vi "Idle Ref Image-Channel ctrls state.vi"() -> ()   [LabVIEW 2020]
uses:
  Typedefs/HW config states enum.ctl
  Typedefs/Channel control synergistic behaviour enum.ctl
  Global Variables/General Globals.vi
  Globals/gl_Windows Ctrl refs.vi
panel:
  out "error out":errorcluster
  in  "error in (no error)":errorcluster
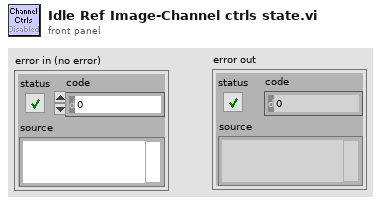
[diagram p1: front panel]
types:
  T1 = typedef "HW config states enum.ctl" = enum16{"Load from file", "Save to file", "Save backup", "Write all", "Read all", "Write XY stage settings", "Write DAQ FPGA settings", "Write Control FPGA settings", "Write Phys Channels", "Write System Config", "Write HW Config", "Save System Config", "Save HW Config", "Clear", "Compare from file"}
  T2 = typedef "Hardware Configuration settings.ctl" = cluster{"Dev. PC":bool, "Swap XY on stage":bool, "No of AOD":u8, "MC Supported":bool, "Axial MC":bool, "Computer MAC address":string, "Externalise Triggers":bool, "Trigger HW config":T3, "DAQmx Chan":T4, "XY stage available":bool, "XY Stage":T5, "Z stage available":bool, "Z Stage config cluster":T6, "Encoder available":bool, "Encoder":T7, "VidRec available":bool, "Cam VidRec":T8, "Laser Power Control HW config":T9, "Laser 1 available":bool, "Laser 1 config cluster":T10, "Prechirper 1 available":bool, "Prechirper 1 config cluster":T11, "Control system.FPGA available?":bool, "Control Sys. HW config":T12, "DAQ FPGA HW Config":T13, "PMT Voltage Range":T17}
  T3 = typedef "Triggers HW config.ctl" = cluster{"Available Device List":i32, "Device Address":string}
  T4 = typedef "DAQmx physical channels cluster.ctl" = cluster{"Pockels AO":tag, "Hard shutter AO":tag, "PMT AOs":tag, "Galvo AOs":tag, "Power meter AI":tag}
  T5 = typedef "XY Stage config cluster.ctl" = cluster{"COM port":refnum<visa-resource-name>, "Baudrate":i32, "Type":string}
  T6 = typedef "Z Stage config cluster.ctl" = cluster{"COM port":refnum<visa-resource-name>, "Baudrate":i32, "Type":string}
  T7 = typedef "Encoder config cluster.ctl" = cluster{"IP address":string, "Port":u16, "Wheel radius (cm)":dbl, "Encoder Trigger":tag}
  T8 = typedef "Cam VidRec HW config setup cluster.ctl" = cluster{"DO flag-Video record":tag, "DO flag-Trial start":tag}
  T9 = typedef "Laser Power Control HW config.ctl" = cluster{"Laser Power Control":string, "Laser Power Modulation Control":enum16{"NI", "FPGA"}}
  T10 = typedef "Laser 1 config cluster.ctl" = cluster{"COM port":refnum<visa-resource-name>, "Baud Rate":i32, "Type":string}
  T11 = typedef "PreChirper 1 config cluster.ctl" = cluster{"Type":string, "Baud Rate":i32, "COM port":refnum<visa-resource-name>}
  T12 = typedef "Control Sys HW config cluster.ctl" = cluster{"Control system.FPGA Type":enum16{"Virtex 5", "Virtex 7"}, "Control system.Network adapter name":string, "Control system.MAC address":string, "Control system.Ethernet Port":u32, "Control system.Ethernet Port Opened":bool}
  T13 = typedef "DAQ FPGA HW config cluster.ctl" = cluster{"FGPA Ref":T14, "Target":T15, "input card type":T16}
  T14 = typedef "FPGA Ref.ctl" = refnum<k20>
  T15 = typedef "nirio_resource_hc.ctl" = tag
  T16 = typedef "FPGA input type AC-DC.ctl" = enum16{"AC Card", "DC Card"}
  T17 = typedef "PMT Voltage Range.ctl" = cluster{"PMT Voltage Lower Limit":dbl, "PMT Voltage Upper Limit":dbl}
  T18 = typedef "Channel control synergistic behaviour enum.ctl" = enum16{"Left disabled-Right enabled", "Left enabled-Right disabled", "Both enabled"}
  T19 = typedef "Live window-ctrl refs.ctl" = cluster{"This VI":refnum<vi>, "Pane":refnum<vi>, "Show REF Image Left":refnum<vi>, "Show REF Image Right":refnum<vi>, "Snapshot":refnum<vi>, "Left Image Palette":refnum<vi>, "Right Image Palette":refnum<vi>, "Left Channel":refnum<vi>, "Right Channel":refnum<vi>, "Left image intensity":refnum<vi>, "Right image intensity":refnum<vi>, "Left Image Display":T20, "Right Image Display":T20, "Refresh rate ind (Hz)":refnum<vi>, "Acq rate ind (Hz)":refnum<vi>, "Stop (ind)":refnum<vi>}
  T20 = typedef "Image display ref.ctl" = refnum<vi>
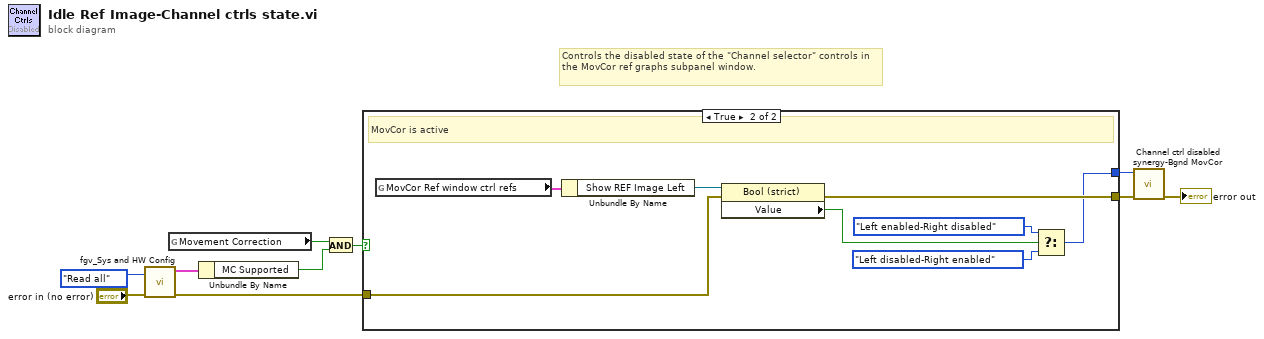
[diagram p0: block diagram]
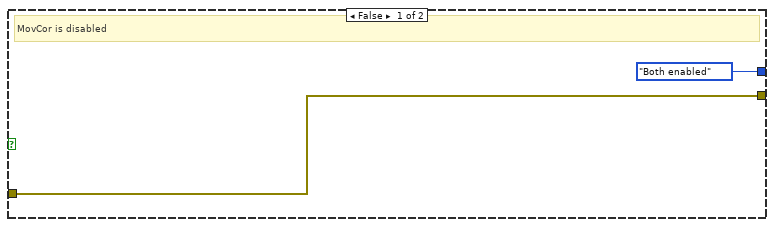
[diagram p2: hidden frame]
diagram:
  # "Controls the disabled state of the \"Channel selector\" controls in the MovCor ref graphs subpanel window."
  n1 = call "fgv_Sys and HW Config.vi"("Function"=HW_config_states_enum."Read all", "error in (no error)"="error in (no error)") -> ("error out"=w5:errorcluster, "Hardware Configuration OUT"=w10:T2)  [unwired: 7 in, 1 out]
  n2 = global read "General Globals.vi" "Movement Correction"() -> (w7:bool)
  n3 = Unbundle By Name(w10) -> ("MC Supported"=w8:bool)
  n4 = And(x=w7, y=w8) -> (x .and. y?=w4:bool)
  n5 = case shown="True" w4 {
    tunnel: w5 -> [w11 w19]
    tunnel: [w11 w18] -> w3
    tunnel: [Channel_control_synergistic_behaviour_enum."Both enabled" ("Behaviour") w16] -> w1
    frame False {
      # "MovCor is disabled"
    }
    frame True {
      # "MovCor is active"
      n6 = global read "gl_Windows Ctrl refs.vi" "MovCor Ref window ctrl refs"() -> (w13:T19)
      n7 = Unbundle By Name(w13) -> ("Show REF Image Left"=w20:refnum<vi>)
      n8 = property on="Property Node" class="Bool (strict)"(reference=w20, error in=w19) -> (error out=w18:errorcluster, "Value"=w17:bool)  [unwired: 1 out]
      n9 = Select(t=Channel_control_synergistic_behaviour_enum."Left enabled-Right disabled" ("Behaviour"), s=w17, f=Channel_control_synergistic_behaviour_enum."Left disabled-Right enabled" ("Behaviour")) -> (s? t:f=w16:T18)
    }
  }
  n10 = call "Channel ctrl disabled synergy-Bgnd MovCor.vi"("error in (no error)"=w3, "Behaviour"=w1) -> ("error out"=→"error out":errorcluster)  [unwired: 9 in]
